vi "gui.vi"(8 "error in (no error)":errorcluster) -> (0 "error out":errorcluster)   [LabVIEW 2018]
uses:
  scope settings.ctl
  PLL param interface.ctl
  <vilib>/Utility/error.llb/Error Cluster From Error Code.vi
  <vilib>/rvi/errors/niLvFpgaAdjustHostInterfaceError.vi
  <vilib>/rvi/interface/nirviReadWriteControl/nirviReadWriteControl.xnode
  <vilib>/rvi/interface/nirviMethod/nirviMethod.xnode
  NiFpgaLv.dll
  <vilib>/rvi/interface/Simulation/niFpgaSimulationCallBeginRW.vi
  <vilib>/rvi/errors/niLvFpgaMergeErrorWithErrorCode.vi
  <vilib>/FPGAPlugInAG/Dynamic/niLvFpga_ReadFifo_Dynamic.vi
panel:
  in  "error in (no error) 2":errorcluster
  in  "exit":bool=TRUE
  out "Time Graph":cluster{"X":dbl, "Y":dbl}[](graph)
  out "Frequency Graph":cluster{"X":dbl, "Y":dbl}[](graph)
  out "error fifo \ncheck #E":errorcluster
  in  "run":bool=TRUE
  in  "decimate":u16=1 min=1
  in  "Analoge In Settings":T1={"gain 1"=1.0, "range 1"=enum."+/- 1 V", "gain 2"=3.0, "range 2"=enum."+/- 1 V"}
  in  "PLL diode":T2={"f21 (kHz)"=20.0, "f43 (kHz)"=32.0, "f32 (kHz)"=68.0, "P gain"=2000.0, "I gain"=5.0, "LP BW (kHz)"=5.0, "notch BW (kHz)"=2.0}
  out "PLL2 freq":T3={"f21 (kHz)"=10.0, "f43 (kHz)"=16.0, "f32 (kHz)"=34.0}
  in  "Lockin":cluster{"LP BW (kHz)":dbl, "notch BW (kHz)":dbl}={"LP BW (kHz)"=1.0, "notch BW (kHz)"=11.0}
  in  "PLL RF mixer":T4={"P gain"=200.0, "I gain"=0.2, "LP BW (kHz)"=1.0, "notch BW (kHz)"=2.0}
  in  "scope settings":T5
  out "PLL1 status":T6={"df1 (Hz)"=-0.0625, "df3 (Hz) "=0.1875, "df2 (Hz)"=-0.1875, "dp1 (deg)"=2.3785400390625, "dp3  (deg)"=1.2744140625, "dp2 (deg)"=1.7633056640625}
  out "PLL2 status":T6={"df1 (Hz)"=0.15625, "df3 (Hz) "=0.15625, "df2 (Hz)"=0.0, "dp1 (deg)"=3.175048828125, "dp3  (deg)"=3.22998046875, "dp2 (deg)"=2.2686767578125}
  out "Lockin status":T7={"pos1 (um)"=4736.829896278072, "pos3 (um)"=-9658.78711345653, "pos2 (um)"=-40902.54137145056} {"pos2 (um)" format="%.3g"; "pos3 (um)" format="%.3g"; "pos1 (um)" format="%.3g"}
  in  "zero phase":bool
  out "pixel counter":i16=100
  out "curr state":T8(ring)
  # "<df> (Hz)"
  # "<|p|> (deg)"
  # "<df> (Hz)"
  # "<|p|> (deg)"
  # "unwr. phase (rad)"
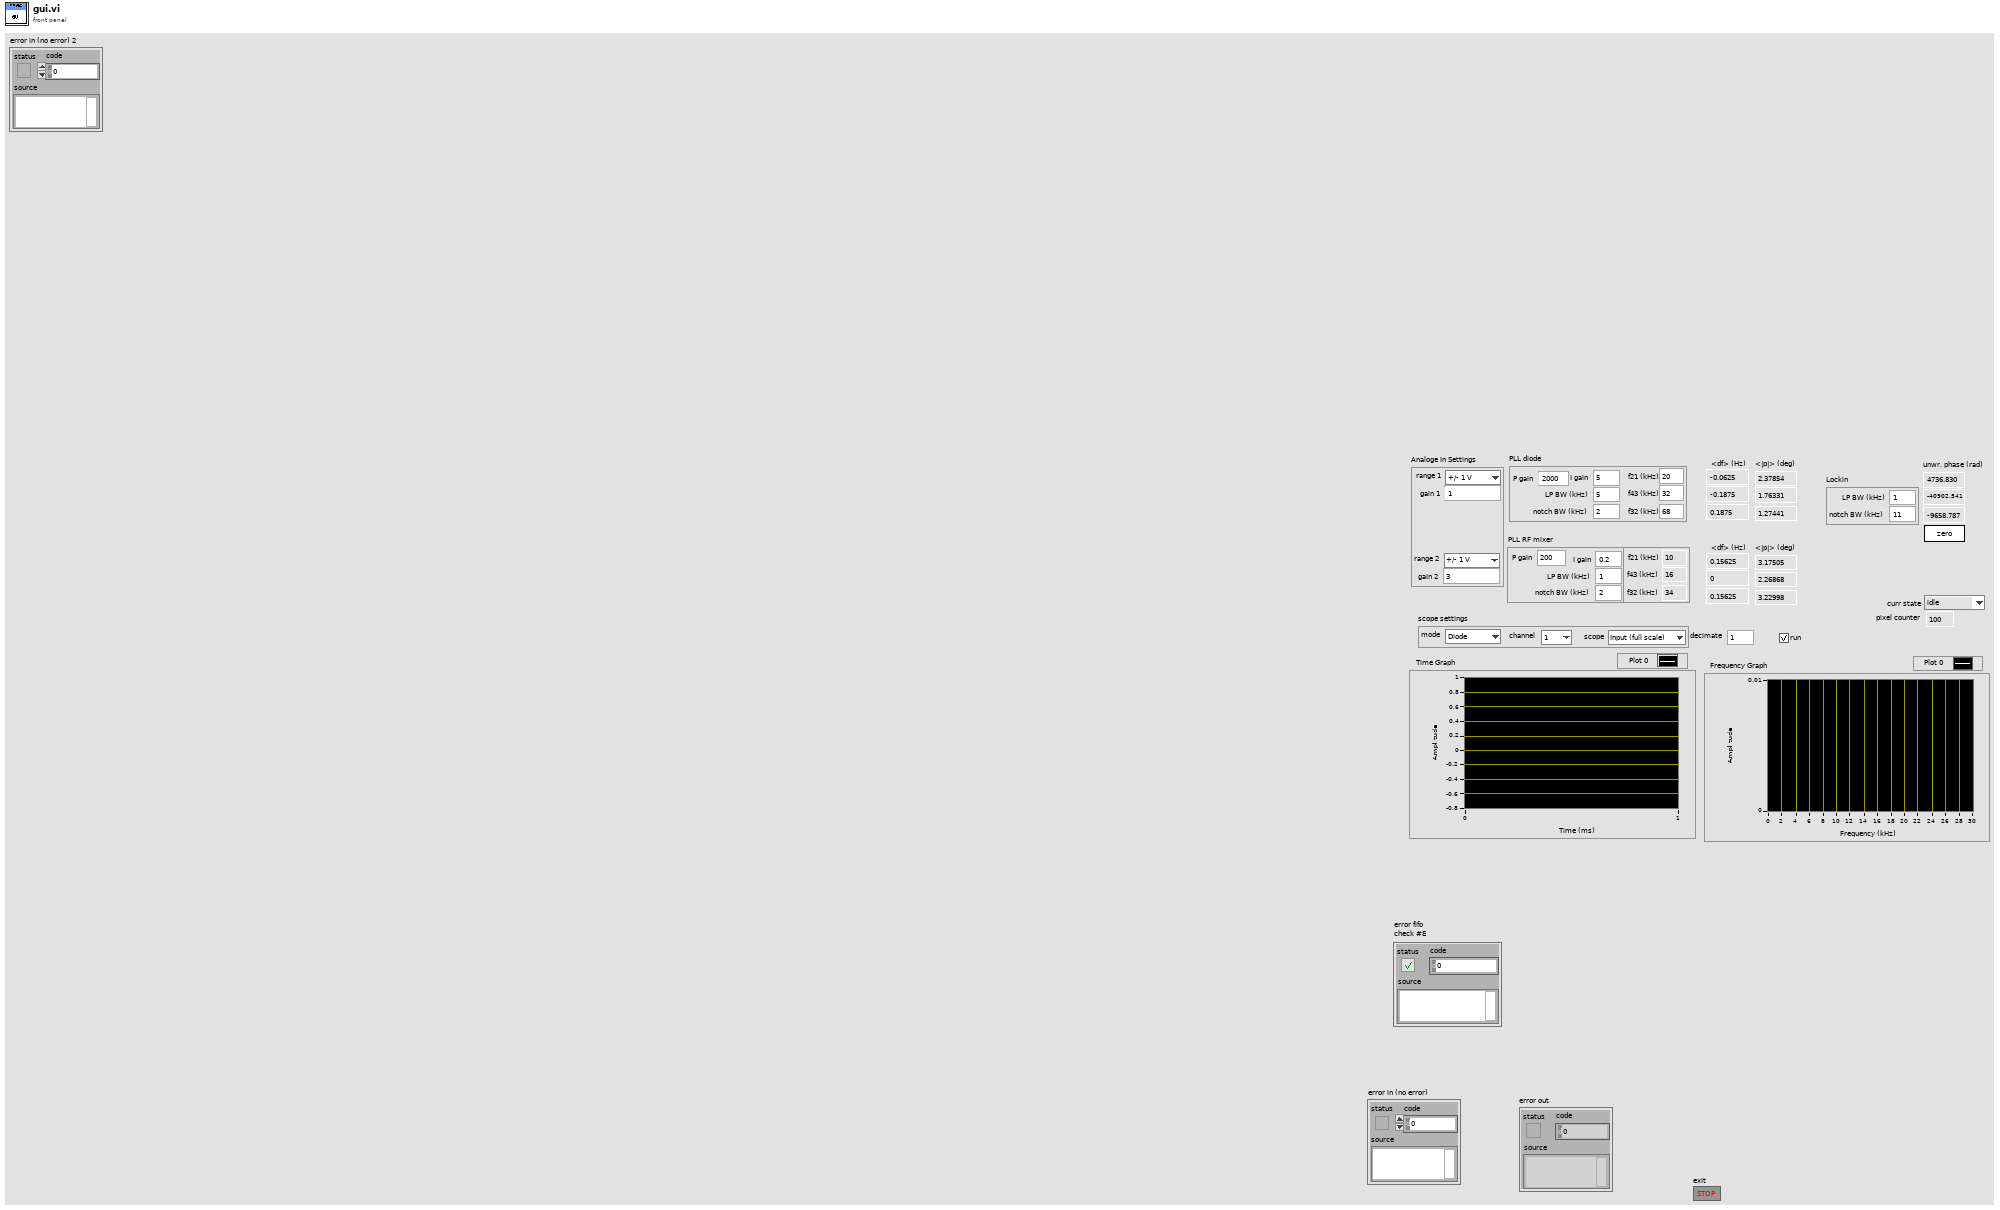
[diagram p1: front panel]
types:
  T1 = cluster{"gain 1":dbl, "range 1":enum16{"+/- 10 V", "+/- 5 V", "+/- 2 V", "+/- 1 V"}, "gain 2":dbl, "range 2":enum16{"+/- 10 V", "+/- 5 V", "+/- 2 V", "+/- 1 V"}}
  T2 = typedef "PLL param interface.ctl" = cluster{"f21 (kHz)":dbl, "f43 (kHz)":dbl, "f32 (kHz)":dbl, "P gain":dbl, "I gain":dbl, "LP BW (kHz)":dbl, "notch BW (kHz)":dbl}
  T3 = cluster{"f21 (kHz)":dbl, "f43 (kHz)":dbl, "f32 (kHz)":dbl}
  T4 = cluster{"P gain":dbl, "I gain":dbl, "LP BW (kHz)":dbl, "notch BW (kHz)":dbl}
  T5 = typedef "scope settings.ctl" = cluster{"mode":enum16{"Diode", "RF mixer", "lockin"}, "channel":enum16{"1", "2", "3"}, "scope":enum16{"Input (full scale)", "PLL out", "Phase error (deg)", "Freq. error (Hz)"}}
  T6 = cluster{"df1 (Hz)":dbl, "df3 (Hz) ":dbl, "df2 (Hz)":dbl, "dp1 (deg)":dbl, "dp3  (deg)":dbl, "dp2 (deg)":dbl}
  T7 = cluster{"pos1 (um)":dbl, "pos3 (um)":dbl, "pos2 (um)":dbl}
  T8 = enum16{"idle", "pre-line", "pre-pixel", "pixel-integration", "pixel-readout", "post-pixel", "post-line"}
  T9 = cluster{"gain ch1":fxp<+,18,6>, "Voltage Range ch1":enum8{"+/- 10 V", "+/- 5 V", "+/- 2 V", "+/- 1 V"}, "gain ch2":fxp<+,18,6>, "Voltage Range ch1 2":enum8{"+/- 10 V", "+/- 5 V", "+/- 2 V", "+/- 1 V"}}
  T10 = cluster{"base freq (Hz)":fxp<+,17,17>[], "P gain":fxp<+,14,14>[], "I gain":fxp<+,20,6>[], "LP1 coeffs":i32[], "scope on":bool, "scope channel":u8, "scope signal":u8, "notch coeffs":i32[]}
  T11 = cluster{"harmonic":fxp<+,20,6>[], "LP1 coeffs":i32[], "scope on":bool, "scope channel":u8, "scope signal":u8}
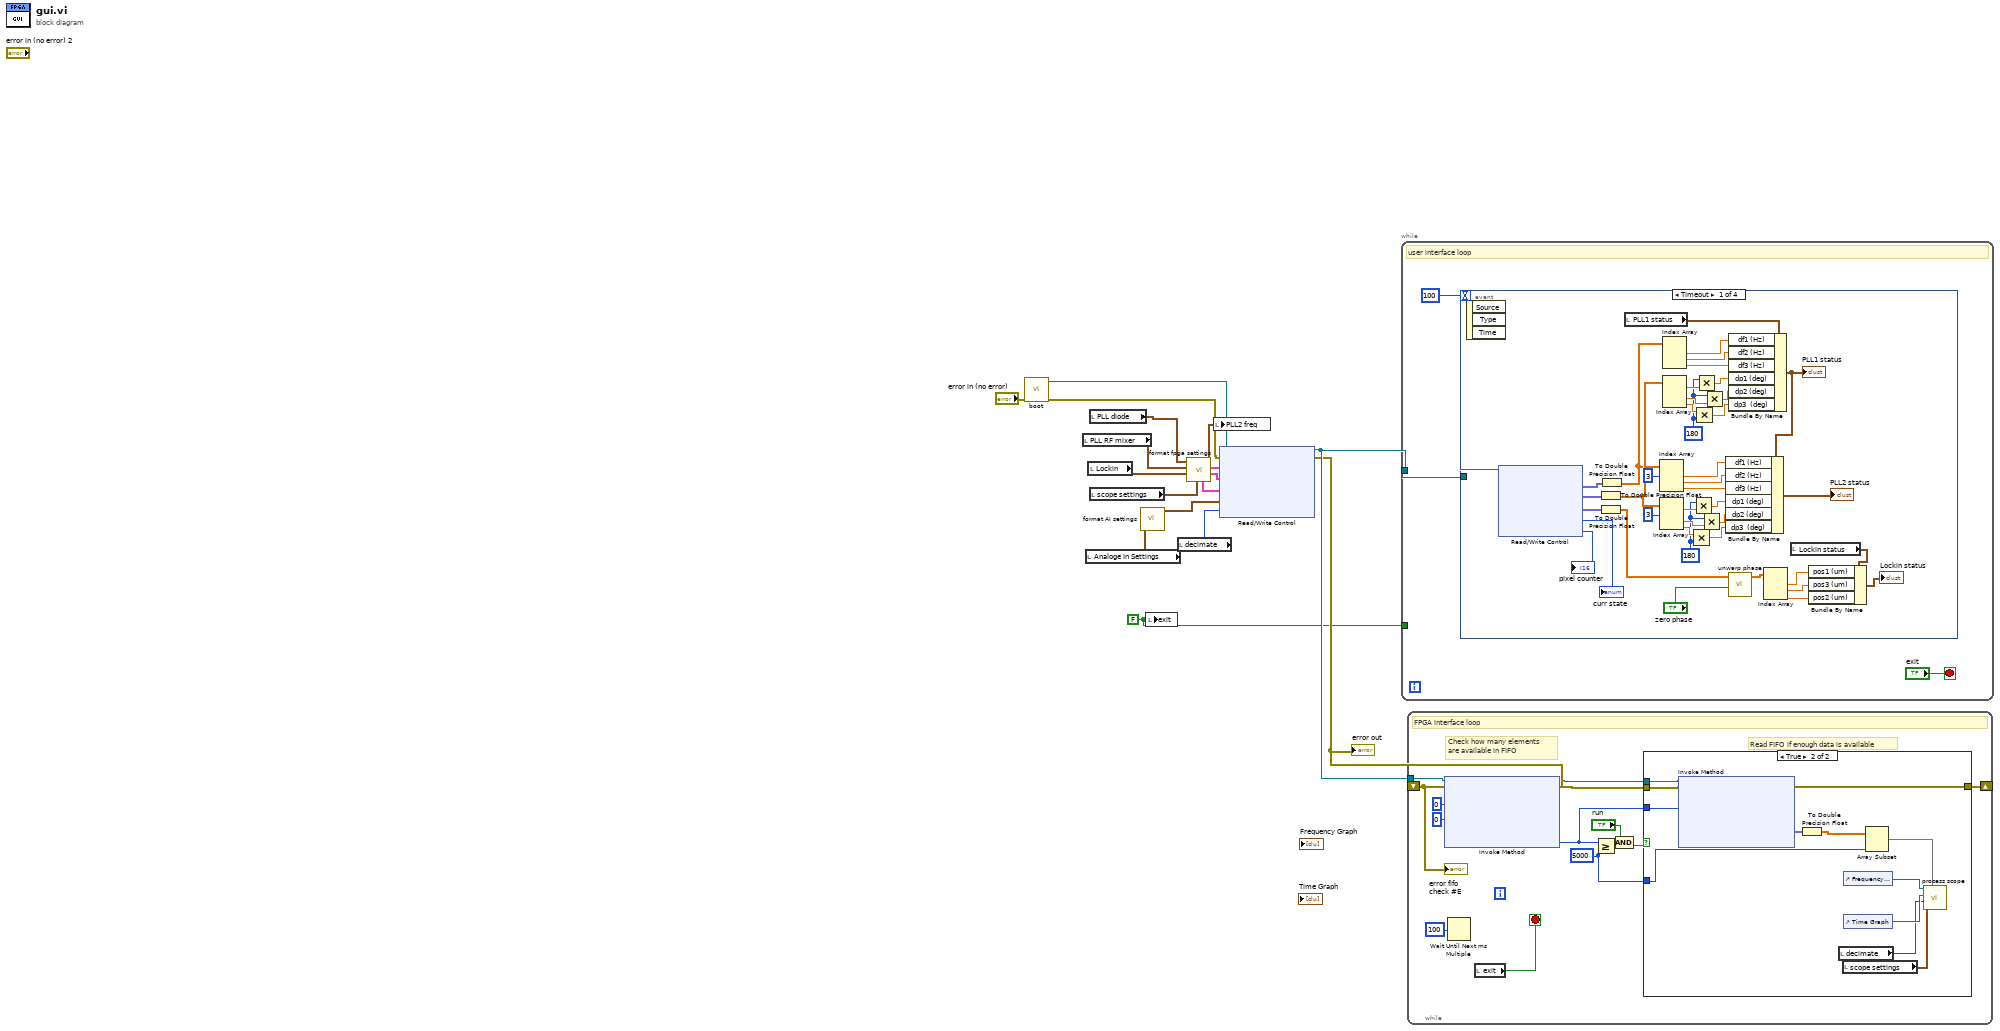
[diagram p0: block diagram]
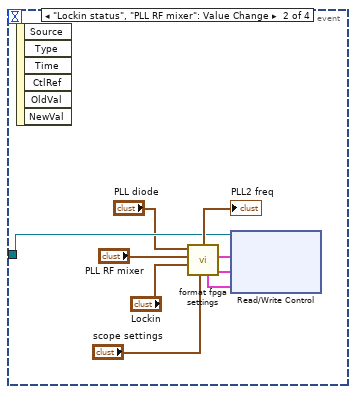
[diagram p3: hidden frame]
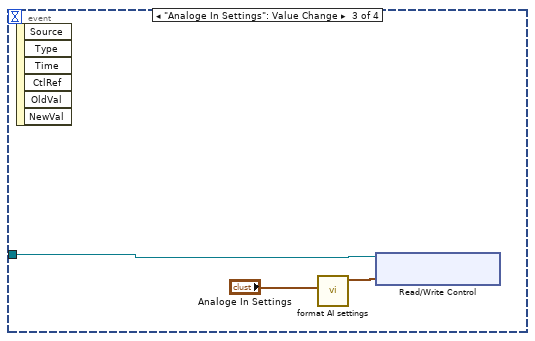
[diagram p4: hidden frame]
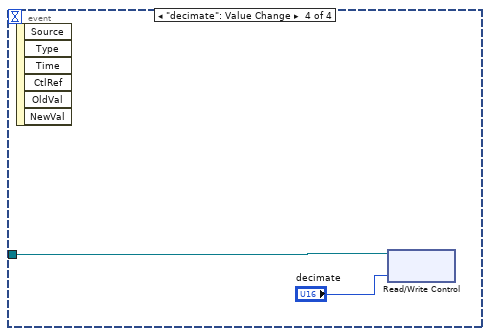
[diagram p5: hidden frame]
diagram:
  w4 = FALSE ("exit")
  n1 = call "boot.vi"("error in (no error)"="error in (no error)") -> ("error out"=w3:errorcluster, "FPGA VI Reference Out"=w2:refnum<k20>)  [unwired: 9 in]
  n2 = local read "PLL RF mixer"() -> (w12:T4)
  n3 = local read "Analoge In Settings"() -> (w8:T1)
  n4 = local read "Lockin"() -> (w13:cluster{"LP BW (kHz)":dbl, "notch BW (kHz)":dbl})
  n5 = local read "PLL diode"() -> (w11:T2)
  n6 = local read "scope settings"() -> (w14:T5)
  n7 = call "format AI settings.vi"("Analoge In Settings"=w8) -> ("analogue in settings (for type) out"=w9:T9)  [unwired: 10 in]
  n8 = local write "exit"(w4) -> ()
  n9 = local read "decimate"() -> (w7:u16)
  n10 = call "format fpga settings.vi"("scope settings"=w14, "Lockin"=w13, "PLL RF mixer"=w12, "PLL diode"=w11) -> ("param PLL2"=w16:T10, "param PLL2 2"=w17:T10, "Cluster"=w10:cluster{dbl, dbl, dbl}, "param Lockin"=w15:T11)  [unwired: 4 in]
  n11 = local write "PLL2 freq"(w10) -> ()
  n12 = xnode "Read/Write Control"("FPGA VI Reference In"=w2, "error in"=w3, "param PLL1"=w17, "param PLL2"=w16, "param Lockin"=w15, "analogue in settings"=w9, "decimate"=w7) -> ("FPGA VI Reference Out"=w6:refnum<k20>, "error out"=w5:errorcluster)
  "error out" <- w5
  n13 = while {
    tunnel: w6 -> [w20]
    tunnel: w4 -> [_]
    stop <- "exit" stop-if-true
    # "user interface loop"
    n14 = event shown="[0] Timeout" {
      selector: _ -> [_ _ _ _]
      dyn-events: _ -> [_ _ _ _]
      timeout: 100 -> [_ _ _ _]
      tunnel: w20 -> [w61 w69 w73 w75]
      event Timeout {
        w38 = 180
        w48 = 180
        n15 = event-data() -> ()  [unwired: 1 in, 3 out]
        n16 = xnode "Read/Write Control"("FPGA VI Reference In"=w61) -> ("freq error mean"=w59:fxp<+/-,16,11>[], "phase error mean"=w55:fxp<+,16,1>[], "phases out"=w31:fxp<+,26,12>[], "curr state"=→"curr state":T8, "pixel counter"=→"pixel counter":i16)  [unwired: 1 in, 2 out]
        n17 = To Double Precision Float(number=w55) -> (double precision float=w36:dbl[])
        n18 = To Double Precision Float(number=w31) -> (double precision float=w24:dbl[])
        n19 = To Double Precision Float(number=w59) -> (double precision float=w35:dbl[])
        n20 = local read "PLL1 status"() -> (w60:T6)
        n21 = Index Array(array=w35, index #1=3 ("index")) -> (element #1=w47:dbl, element #2=w46:dbl, element #3=w45:dbl)  [unwired: 2 in]
        n22 = Index Array(array=w36, index #1=3 ("index")) -> (element #1=w39:dbl, element #2=w43:dbl, element #3=w44:dbl)  [unwired: 2 in]
        n23 = Index Array(array=w35) -> (element #1=w58:dbl, element #2=w57:dbl, element #3=w56:dbl)  [unwired: 3 in]
        n24 = Index Array(array=w36) -> (element #1=w49:dbl, element #2=w53:dbl, element #3=w54:dbl)  [unwired: 3 in]
        n25 = Multiply(x=w44, y=w38) -> (x*y=w40:dbl)
        n26 = Multiply(x=w38, y=w39) -> (x*y=w42:dbl)
        n27 = Multiply(x=w54, y=w48) -> (x*y=w50:dbl)
        n28 = Multiply(x=w48, y=w49) -> (x*y=w52:dbl)
        n29 = Multiply(x=w38, y=w43) -> (x*y=w41:dbl)
        n30 = Multiply(x=w48, y=w53) -> (x*y=w51:dbl)
        n31 = Bundle By Name(cluster=w60, "df1 (Hz)"=w58, "df2 (Hz)"=w57, "df3 (Hz)"=w56, "dp1 (deg)"=w52, "dp2 (deg)"=w51, "dp3  (deg)"=w50) -> (w37:T6)
        "PLL1 status" <- w37
        n32 = Bundle By Name(cluster=w37, "df1 (Hz)"=w47, "df2 (Hz)"=w46, "df3 (Hz)"=w45, "dp1 (deg)"=w42, "dp2 (deg)"=w41, "dp3  (deg)"=w40) -> (→"PLL2 status":T6)
        n33 = call "unwarp phase.vi"("zero!"="zero phase", "phase in (0..4096)"=w24) -> ("unwrapped phase out (rad)"=w25:dbl[])  [unwired: 9 in]
        n34 = Index Array(array=w25) -> (element #1=w29:dbl, element #2=w28:dbl, element #3=w27:dbl)  [unwired: 3 in]
        n35 = local read "Lockin status"() -> (w30:T7)
        n36 = Bundle By Name(cluster=w30, "pos1 (um)"=w29, "pos3 (um)"=w28, "pos2 (um)"=w27) -> (→"Lockin status":T7)
      }
      event "Lockin status", "PLL RF mixer": Value Change {
        n37 = event-data() -> ()  [unwired: 1 in, 6 out]
        n38 = call "format fpga settings.vi"("scope settings"="scope settings", "Lockin"="Lockin", "PLL RF mixer"="PLL RF mixer", "PLL diode"="PLL diode") -> ("param PLL2"=w67:T10, "param PLL2 2"=w68:T10, "Cluster"=→"PLL2 freq":cluster{dbl, dbl, dbl}, "param Lockin"=w66:T11)  [unwired: 4 in]
        n39 = xnode "Read/Write Control"("FPGA VI Reference In"=w69, "param PLL1"=w68, "param PLL2"=w67, "param Lockin"=w66) -> ()  [unwired: 1 in, 2 out]
      }
      event "Analoge In Settings": Value Change {
        n40 = event-data() -> ()  [unwired: 1 in, 6 out]
        n41 = call "format AI settings.vi"("Analoge In Settings"="Analoge In Settings") -> ("analogue in settings (for type) out"=w72:T9)  [unwired: 10 in]
        n42 = xnode "Read/Write Control"("FPGA VI Reference In"=w73, "analogue in settings"=w72) -> ()  [unwired: 1 in, 2 out]
      }
      event "decimate": Value Change {
        n43 = event-data() -> ()  [unwired: 1 in, 6 out]
        n44 = xnode "Read/Write Control"("FPGA VI Reference In"=w75, "decimate"="decimate") -> ()  [unwired: 1 in, 2 out]
      }
    }
  }
  n45 = while {
    tunnel: w6 -> [w89]
    shift-right: [w81] -> _
    shift-left: w5 -> [w80]
    stop <- w76 stop-if-true
    w79 = u32 5000 ("y")
    # "Read FIFO if enough data is available"
    # "Check how many elements\nare available in FIFO"
    # "FPGA interface loop"
    n46 = xnode "Invoke Method"("FPGA VI Reference In"=w89, "error in"=w80, "Number of Elements"=u32 0, "Timeout (ms)"=0) -> ("FPGA VI Reference Out"=w85:refnum<k20>, "error out"=w82:errorcluster, "Elements Remaining"=w84:u32)  [unwired: 1 out]
    n47 = Wait Until Next ms Multiple(millisecond multiple=u32 100) -> ()  [unwired: 1 out]
    n48 = local read "exit"() -> (w76:bool)
    n49 = Greater Or Equal?(x=w84, y=w79) -> (x >= y?=w83:bool)
    n50 = And(x="run", y=w83) -> (x .and. y?=w78:bool)
    n51 = case shown="True" w78 {
      tunnel: w85 -> [_ w102]
      tunnel: w84 -> [_ w101]
      tunnel: w82 -> [w90 w99]
      tunnel: [w90 w98] -> w81
      tunnel: w79 -> [_ w97]
      frame False {
      }
      frame True {
        n52 = xnode "Invoke Method"("FPGA VI Reference In"=w102, "error in"=w99, "Number of Elements"=w101) -> ("error out"=w98:errorcluster, "Data"=w100:fxp<+/-,16,1>[])  [unwired: 1 in, 2 out]
        n53 = To Double Precision Float(number=w100) -> (double precision float=w96:dbl[])
        n54 = local read "decimate"() -> (w92:u16)
        n55 = local read "scope settings"() -> (w91:T5)
        n56 = control-ref of="Frequency Graph"() -> (w94:refnum<vi>)
        n57 = control-ref of="Time Graph"() -> (w93:refnum<vi>)
        n58 = Array Subset(array=w96, length=w97) -> (w95:dbl[])  [unwired: 1 in]
        n59 = call "process scope.vi"("data in"=w95, "scope settings"=w91, "decimate"=w92, "Time Graph"=w93, "Frequency Graph"=w94) -> ()  [unwired: 7 in]
      }
    }
    "error fifo \ncheck #E" <- w80
  }
